vi "SV Update Signal.vi"(0 "current configuration":refnum<class "SV Signal.lvclass">, 5 "new configuraiton":refnum<class "SV Function.lvclass">, 11 "error in (no error)":errorcluster) -> (4 "updated configuration":refnum<class "SV Function.lvclass">, 15 "error out":errorcluster)   [LabVIEW 2017, in "SV Function.lvclass"]
uses:
  <vilib>/addons/_NISVFA/_Generation/Signal Generation/SV Function/SV Function.lvclass
  <vilib>/addons/_NISVFA/_Generation/Signal Generation/SV Signal/SV Signal.lvclass
  C:/Program Files (x86)/National Instruments/LabVIEW 2017/vi.lib/addons/_NISVFA/_Generation/Signal Generation/SV Signal/SV Signal.lvclass
  <vilib>/addons/_NISVFA/_Generation/Signal Generation/SV Signal/sv_Signal State Attribute.ctl
  <vilib>/addons/_NISVFA/_Generation/Signal Generation/SV Function/SV Function.lvclass/SV Function.ctl
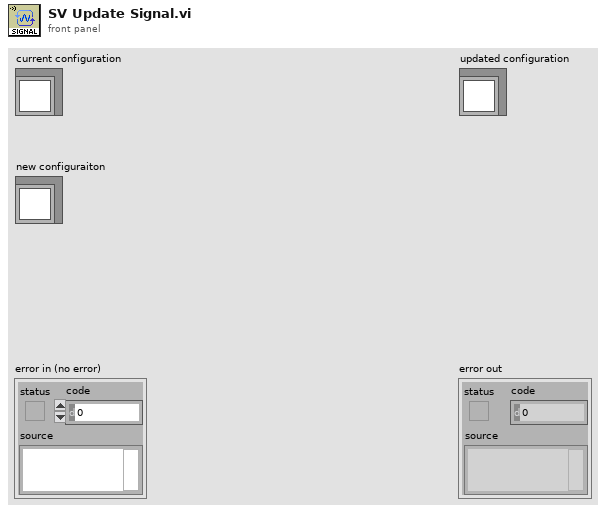
[diagram p1: front panel]
types:
  T1 = typedef "SV Signal.lvclass/sv_Signal State Attribute.ctl" = string
  T2 = typedef "SV Signal.lvclass/sv_System Timing Model.ctl" = i64
  T3 = typedef "SV Signal.lvclass/sv_Generation State.ctl" = enum16{"Idle", "Ramp Up", "Pre-Measurement Settling", "Measurement", "Post-Measurement Settling", "Discrete Sweep Transition", "Ramp Down", "Update"}
  T4 = cluster{"system timing model":T2, "state":cluster{"RESET":bool, "generator timestamp":timestamp, "elapsed seconds":dbl, "elapsed samples":u64, "generation state":T3, "time offset at state":dbl, "samples generated at state":u64, "signal state":variant}, "duration of state":dbl, "samples remaining at state":i32}
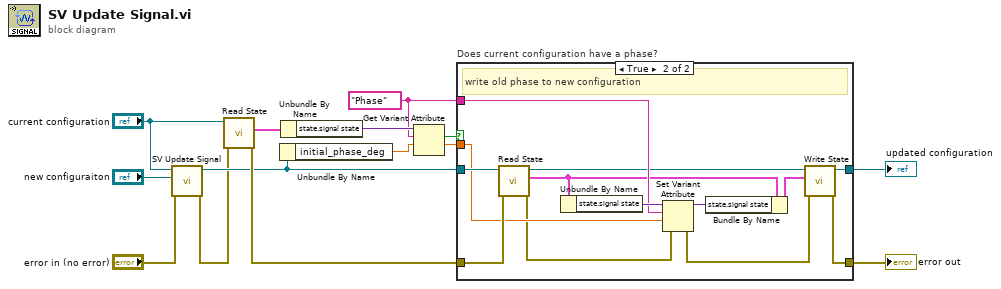
[diagram p0: block diagram]
diagram:
  w7 = T1 "Phase" ("attribute")
  n1 = call-parent "SV Update Signal.vi"("current configuration"="current configuration", "new configuration"="new configuraiton", "error in (no error)"="error in (no error)") -> ("updated configuration"=w4:refnum<class "SV Function.lvclass">, "error out"=w1:errorcluster)  [unwired: 11 in]
  n2 = call <vilib>:"Read State.vi"("error in (no error)"=w1, "signal configuration"="current configuration") -> ("error out"=w6:errorcluster, "generator state"=w14:T4)  [unwired: 7 in, 1 out]
  n3 = Unbundle By Name(w4) -> ("initial_phase_deg"=w12:dbl)
  n4 = Unbundle By Name(w14) -> ("state.signal state"=w13:variant)
  n5 = Get Variant Attribute(Variant=w13, name=w7, default value (empty Variant)=w12) -> (found=w9:bool, value=w8:dbl)  [unwired: 1 in, 2 out]
  n6 = case "Does current configuration have a phase?" shown="True" w9 {
    tunnel: w4 -> [w16 w29]
    tunnel: w6 -> [w15 w28]
    tunnel: [w16 w22] -> w11
    tunnel: [w15 w20] -> w10
    tunnel: w8 -> [_ w19]
    tunnel: w7 -> [_ w26]
    frame False {
      # "No phase exists to write to new configuration"
    }
    frame True {
      # "write old phase to new configuration"
      n7 = call <vilib>:"Read State.vi"("error in (no error)"=w28, "signal configuration"=w29) -> ("error out"=w18:errorcluster, "generator state"=w25:T4, "signal configuration"=w23:refnum<class "SV Function.lvclass">)  [unwired: 7 in]
      n8 = Unbundle By Name(w25) -> ("state.signal state"=w27:variant)
      n9 = Set Variant Attribute(Variant=w27, name=w26, value=w19, error in=w18) -> (Variant out=w24:variant, error out=w17:errorcluster)  [unwired: 1 out]
      n10 = Bundle By Name(cluster=w25, "state.signal state"=w24) -> (w21:T4)
      n11 = call <vilib>:"Write State.vi"("error in (no error)"=w17, "generator state"=w21, "signal configuration"=w23) -> ("error out"=w20:errorcluster, "signal configuration"=w22:refnum<class "SV Function.lvclass">)  [unwired: 7 in]
    }
  }
  "error out" <- w10
  "updated configuration" <- w11
